vi "SetParam.vi"(8 "error in (no error)":errorcluster caption="entrée d'erreur (pas d'erreur)", 10 "label_binarize":T1={"classes"=[], "neg_label"=0, "pos_label"=1, "sparse_output"=FALSE}, 11 "label_binarize.lvclass":refnum<class "label_binarize.lvclass">) -> (0 "error out":errorcluster caption="sortie d'erreur", 3 "label_binarize.lvclass":refnum<class "label_binarize.lvclass">)   [LabVIEW 2020, in "label_binarize.lvclass"]
doc: "Set Parameters"
uses:
  label_binarize.lvclass
  label_binarize.lvclass/label_binarize.ctl
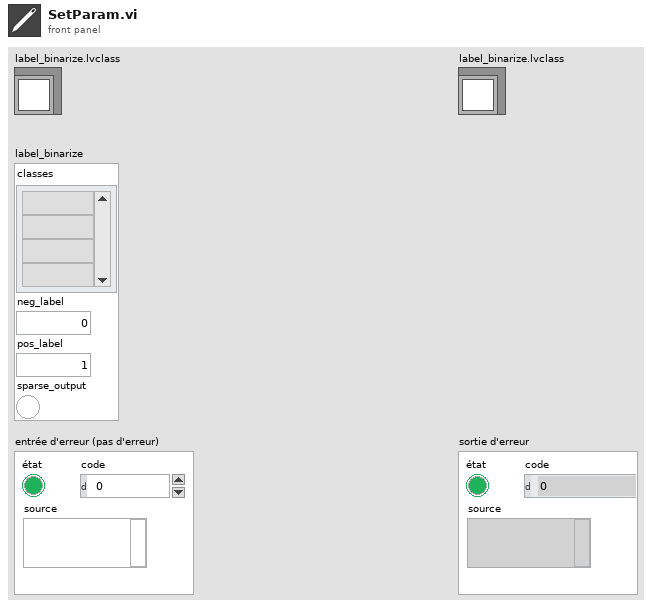
[diagram p1: front panel]
types:
  T1 = cluster{"classes":string[][], "neg_label":i32, "pos_label":i32, "sparse_output":bool}
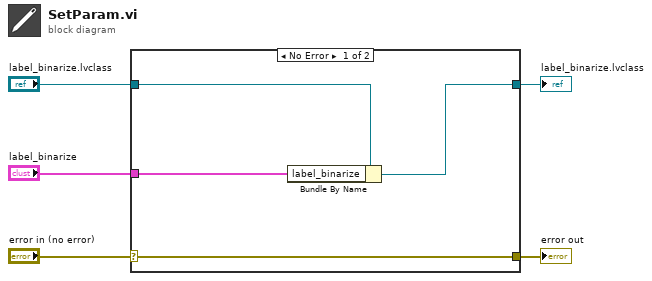
[diagram p0: block diagram]
diagram:
  n1 = case shown="No Error" "error in (no error)" {
    selector: "error in (no error)" -> [w9 w10]
    tunnel: [w9 w10] -> w4
    tunnel: [w7 w11] -> w2
    tunnel: "label_binarize.lvclass" -> [w8 w11]
    tunnel: "label_binarize" -> [w6 _]
    frame No Error {
      n2 = Bundle By Name(cluster=w8, "label_binarize"=w6) -> (w7:refnum<class "label_binarize.lvclass">)
    }
    frame Error {
    }
  }
  "error out" <- w4
  "label_binarize.lvclass" <- w2
